vi "busy_wait_embed.vi"(7 "callee":refnum<vi>, 8 "error in (no error)":errorcluster, 10 "configuration":T2={"dialog_text"="", "wait_s"=0.0, "inner_color"=16711680, "outer_color"=6618880, "knob_reference"=refnum, "dialog_reference"=refnum, "event_registration"=refnum}, 11 "v1 in":refnum<class "v1.lvclass">) -> (0 "error out":errorcluster, 2 "dialog_selection":T1, 3 "v1 out":refnum<class "v1.lvclass">)   [LabVIEW 2015, in "lv-dialog.lvlib" / "v1.lvlib" / "v1.lvclass"]
doc: "The busy/wait api can be used to provide feedback when a process is going to take a long time, as implemented within the base api class, it doesn't have a lot of functional feedback aside from setting or unsetting busy. The configuration provides a time (in seconds), the dialog message as well as an event registration that can be used to indicate \"done\" from the outside.\n\nThis is implemented by the base api class (not the embedded) by using the \"Set Busy\" and \"Unset Busy\" VIs."
uses:
  v1.lvclass
  _controls/selection.ctl
  _controls/error.ctl
  lv-dialog.lvlib
  v1.lvlib
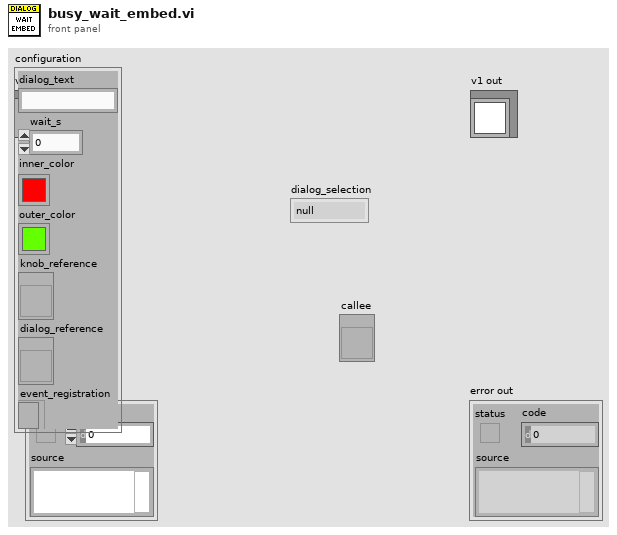
[diagram p1: front panel]
types:
  T1 = typedef "lv-dialog.lvlib/v1.lvlib/selection.ctl" = enum16{"null", "panel_closed", "button_1", "button_2", "button_3", "cancelled"}
  T2 = cluster{"dialog_text":string, "wait_s":dbl, "inner_color":u32, "outer_color":u32, "knob_reference":refnum<vi>, "dialog_reference":refnum<vi>, "event_registration":refnum<event-registration>}
  T3 = typedef "lv-dialog.lvlib/error.ctl" = enum16{"null", "not_implemented"}
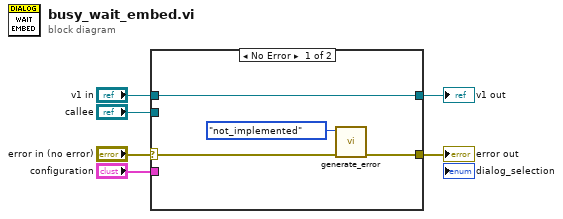
[diagram p0: block diagram]
diagram:
  n1 = case shown="No Error" "error in (no error)" {
    selector: "error in (no error)" -> [w8 w12]
    tunnel: [w7 w12] -> w5
    tunnel: [w10 w11] -> w3
    tunnel: "v1 in" -> [w10 w11]
    tunnel: "callee" -> [_ _]
    tunnel: "configuration" -> [_ _]
    frame No Error {
      n2 = call "generate_error.vi"("error in (no error)"=w8, "error"=error."not_implemented") -> ("error out"=w7:errorcluster)  [unwired: 9 in]
    }
    frame Error {
    }
  }
  "error out" <- w5
  "v1 out" <- w3
